vi "splash_v1.0.vi"() -> ()   [LabVIEW 2025]
doc: "Use this template to build a producer/consumer design pattern with events to produce queue items. Use this design pattern instead of the User Interface Event Handler pattern for user interfaces when you want to execute code asynchronously in response to an event without slowing the user interface responsiveness."
uses:
  <vilib>/Platform/browser.llb/Open URL in Default Browser (string).vi
panel:
  in  "transparency_rate(ms)":i32=25
  in  "close_delay(sec)":dbl=5.0
  out "loading_msg":string="Loading DAQ resources..."
  in  "producer_exit":bool
  # "www.freshconsulting.com"
  # "SLUG DEMO  v1.0.0.6"
  # "Strategy"
  # "Hardware"
  # "Software"
  # "Design"
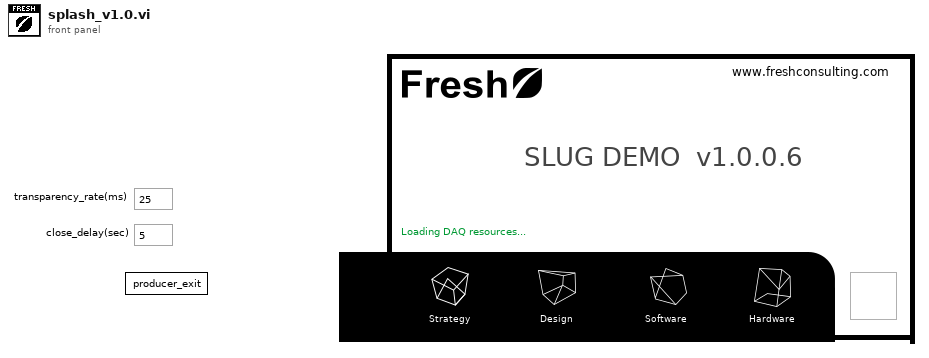
[diagram p1: front panel]
types:
  T1 = enum32{"Invalid", "Standard", "Closed", "Hidden", "Minimized", "Maximized"}
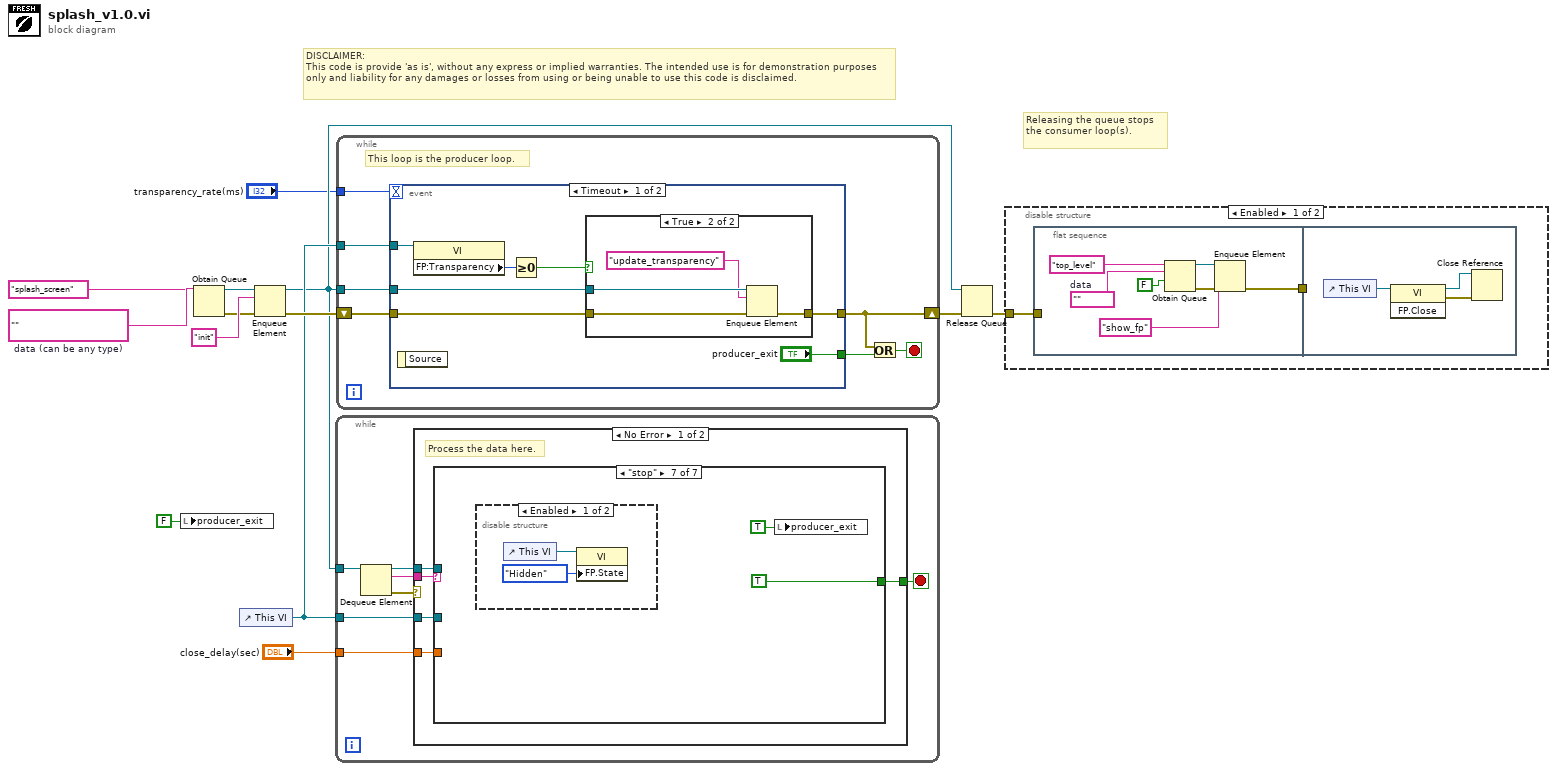
[diagram p0: block diagram]
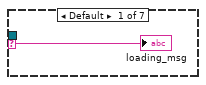
[diagram p3: hidden frame]
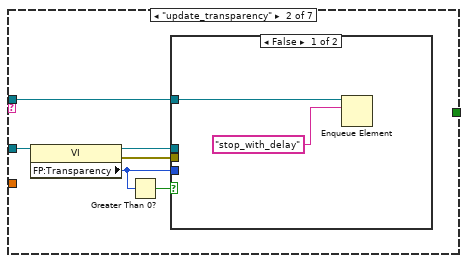
[diagram p4: hidden frame]
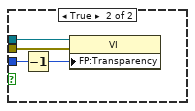
[diagram p5: hidden frame]
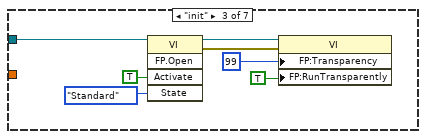
[diagram p6: hidden frame]
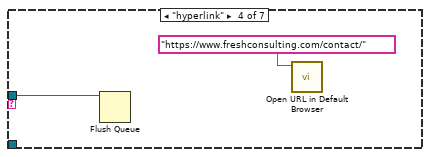
[diagram p7: hidden frame]
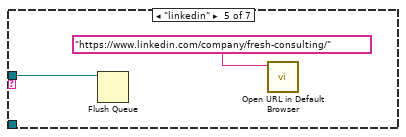
[diagram p8: hidden frame]
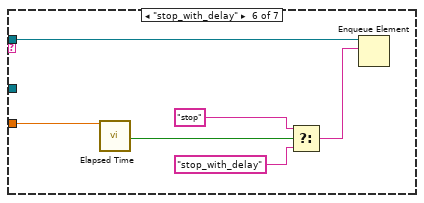
[diagram p9: hidden frame]
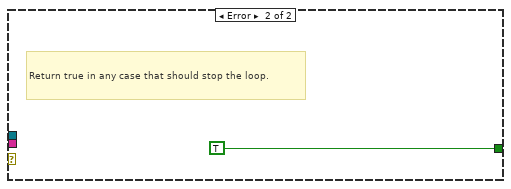
[diagram p11: hidden frame]
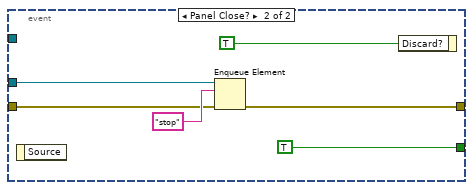
[diagram p13: hidden frame]
diagram:
  w12 = ""  # data (can be any type)
  # "DISCLAIMER:\nThis code is provide 'as is', without any express or implied warranties. The intended use is for demonstration purposes only and liability for any damages or losses from using or being unable to use this code is disclaimed."
  # "Releasing the queue stops the consumer loop(s)."
  n1 = local write "producer_exit"(FALSE ("producer_exit")) -> ()
  n2 = Obtain Queue(name (unnamed)="splash_screen", element data type=w12) -> (queue out=w7:refnum<queue>, error out=w5:errorcluster)  [unwired: 3 in, 1 out]
  n3 = control-ref of="This VI"() -> (w4:refnum<vi>)
  n4 = Enqueue Element(queue=w7, element="init", error in (no error)=w5) -> (queue out=w3:refnum<queue>, error out=w6:errorcluster)  [unwired: 1 in, 1 out]
  n5 = while {
    tunnel: w3 -> [w20]
    tunnel: w4 -> [w15]
    tunnel: "close_delay(sec)" -> [w14]
    stop <- w17 stop-if-true
    n6 = Dequeue Element(queue=w20) -> (queue out=w16:refnum<queue>, element=w18:string, error out=w19:errorcluster)  [unwired: 2 in, 1 out]
    n7 = case shown="No Error" w19 {
      tunnel: w18 -> [w25 _]
      tunnel: [w24 TRUE] -> w17
      tunnel: w16 -> [w23 _]
      tunnel: w15 -> [w22 _]
      tunnel: w14 -> [w21 _]
      frame No Error {
        # "Process the data here."
        n8 = case shown="\"stop\"" w25 {
          selector: w25 -> [w26 _ _ _ _ _ _]
          tunnel: [_ _ _ _ _ _ TRUE] -> w24
          tunnel: w23 -> [_ w27 _ w46 w48 w55 _]
          tunnel: w22 -> [_ w30 w39 _ _ _ _]
          tunnel: w21 -> [_ _ _ _ _ w50 _]
          frame Default {
            "loading_msg" <- w26
          }
          frame "update_transparency" {
            n9 = property class="VI"(reference=w30) -> (reference out=w32:refnum<vi>, error out=w31:errorcluster, "FP:Transparency"=w29:u8)  [unwired: 1 in]
            n10 = Greater Than 0?(x=w29) -> (x > 0?=w28:bool)
            n11 = case shown="False" w28 {
              tunnel: w32 -> [_ w38]
              tunnel: w31 -> [_ w37]
              tunnel: w29 -> [_ w35]
              tunnel: w27 -> [w33 _]
              frame False {
                n12 = Enqueue Element(queue=w33, element="stop_with_delay") -> ()  [unwired: 2 in, 3 out]
              }
              frame True {
                n13 = Decrement(x=w35) -> (x-1=w36:u8)
                n14 = property class="VI"(reference=w38, error in=w37, "FP:Transparency"=w36) -> ()  [unwired: 2 out]
              }
            }
          }
          frame "init" {
            n15 = invoke class="VI" method="FP.Open"(reference=w39, "Activate"=TRUE ("Activate?"), "State"=T1."Standard") -> (reference out=w45:refnum<vi>, error out=w44:errorcluster)  [unwired: 2 in, 3 out]
            n16 = property class="VI"(reference=w45, error in=w44, "FP:Transparency"=u8 99 ("Front Panel Window:Transparency"), "FP:RunTransparently"=TRUE ("Front Panel Window:Run VI Transparently")) -> ()  [unwired: 2 out]
          }
          frame "hyperlink" {
            n17 = Flush Queue(queue=w46) -> ()  [unwired: 1 in, 3 out]
            n18 = call-poly <vilib>:"Open URL in Default Browser.vi"("URL"="https://www.freshconsulting.com/contact/") -> ()  [unwired: 5 in, 2 out]
          }
          frame "linkedin" {
            n19 = Flush Queue(queue=w48) -> ()  [unwired: 1 in, 3 out]
            n20 = call-poly <vilib>:"Open URL in Default Browser.vi"("URL"="https://www.linkedin.com/company/fresh-consulting/") -> ()  [unwired: 5 in, 2 out]
          }
          frame "stop_with_delay" {
            n21 = call "Elapsed Time"("Time Target (s)"=w50) -> ("Time has Elapsed"=w54:bool)  [unwired: 11 in, 7 out]
            n22 = Select(t="stop" ("element"), s=w54, f="stop_with_delay" ("element")) -> (s? t:f=w51:string)
            n23 = Enqueue Element(queue=w55, element=w51) -> ()  [unwired: 2 in, 3 out]
          }
          frame "stop" {
            n24 = disable-structure shown="Enabled" {
              frame Enabled {
                n25 = control-ref of="This VI"() -> (w58:refnum<vi>)
                n26 = property class="VI"(reference=w58, "FP.State"=T1."Hidden" ("Front Panel Window:State")) -> ()  [unwired: 1 in, 2 out]
              }
              frame Disabled {
              }
            }
            n27 = local write "producer_exit"(TRUE ("producer_exit")) -> ()
          }
        }
      }
      frame Error {
        # "Return true in any case that should stop the loop."
      }
    }
  }
  n28 = while {
    shift-right: [w63] -> w13
    shift-left: w6 -> [w66]
    tunnel: w3 -> [w67]
    tunnel: w4 -> [w62]
    tunnel: "transparency_rate(ms)" -> [w61]
    stop <- w64 stop-if-true
    # "This loop is the producer loop."
    n29 = event shown="[0] Timeout" {
      selector: _ -> [_ _]
      dyn-events: _ -> [_ _]
      timeout: w61 -> [_ _]
      tunnel: w67 -> [w73 w84]
      tunnel: w66 -> [w72 w83]
      tunnel: [w71 w82] -> w63
      tunnel: ["producer_exit" TRUE ("stop")] -> w65
      tunnel: w62 -> [w69 _]
      event Timeout {
        n30 = event-data() -> ()  [unwired: 1 in, 1 out]
        n31 = property class="VI"(reference=w69) -> ("FP:Transparency"=w70:u8)  [unwired: 1 in, 2 out]
        n32 = Greater Or Equal To 0?(x=w70) -> (x >= 0?=w68:bool)
        n33 = case shown="True" w68 {
          tunnel: w73 -> [_ w79]
          tunnel: w72 -> [w75 w78]
          tunnel: [w75 w77] -> w71
          frame False {
          }
          frame True {
            n34 = Enqueue Element(queue=w79, element="update_transparency", error in (no error)=w78) -> (error out=w77:errorcluster)  [unwired: 1 in, 2 out]
          }
        }
      }
      event Panel Close? {
        n35 = event-data() -> ()  [unwired: 1 in, 1 out]
        n36 = Enqueue Element(queue=w84, element="stop", error in (no error)=w83) -> (error out=w82:errorcluster)  [unwired: 1 in, 2 out]
        n37 = event-data("Discard?"=TRUE) -> ()  [unwired: 1 in, 1 out]
      }
    }
    n38 = Or(x=w63, y=w65) -> (x .or. y?=w64:bool)
  }
  n39 = Release Queue(queue=w3, error in (no error)=w13) -> (error out=w11:errorcluster)  [unwired: 1 in, 2 out]
  n40 = disable-structure shown="Enabled" {
    disable-tunnel: w11 -> [w87 _]
    frame Enabled {
      n41 = flat-sequence {
        tunnel: w87 -> [_]
        tunnel: [w88] -> w86
        tunnel: w86 -> [_]
        frame #0 {
          w90 = ""  # data
          n42 = Obtain Queue(name (unnamed)="top_level", element data type=w90, create if not found? (T)=FALSE) -> (queue out=w94:refnum<queue>, error out=w93:errorcluster)  [unwired: 2 in, 1 out]
          n43 = Enqueue Element(queue=w94, element="show_fp" ("name (unnamed)"), error in (no error)=w93) -> (error out=w88:errorcluster)  [unwired: 1 in, 2 out]
        }
        frame #1 {
          n44 = control-ref of="This VI"() -> (w95:refnum<vi>)
          n45 = invoke class="VI" method="FP.Close"(reference=w95) -> (reference out=w96:refnum<vi>, error out=w97:errorcluster)  [unwired: 2 in, 1 out]
          n46 = Close Reference(reference=w96, error in (no error)=w97) -> ()  [unwired: 1 out]
        }
      }
    }
    frame Disabled {
    }
  }
